vi "IntervalRand.vi"(11 "Max":dbl) -> (3 "x*y":dbl)   [LabVIEW 2014]
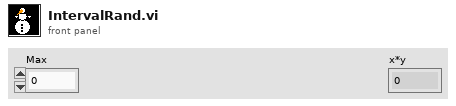
[diagram p1: front panel]
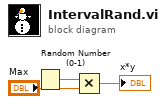
[diagram p0: block diagram]
diagram:
  n1 = Random Number (0-1)() -> (number: 0 to 1=w3:dbl)
  n2 = Multiply(x=w3, y="Max") -> (x*y=→"x*y":dbl)
